vi "Path to Class.vi"(8 "error in (no error)":errorcluster) -> (0 "error out":errorcluster, 3 "Usuarios out":refnum<class "Usuarios.lvclass">)   [LabVIEW 2019, in "Usuarios.lvclass"]
uses:
  Usuarios.lvclass
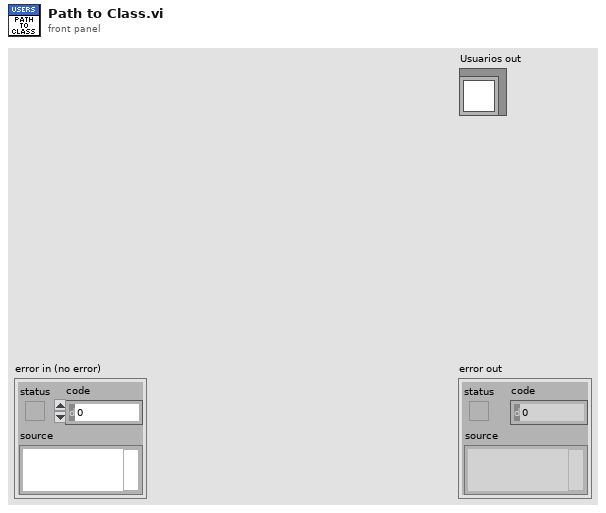
[diagram p1: front panel]
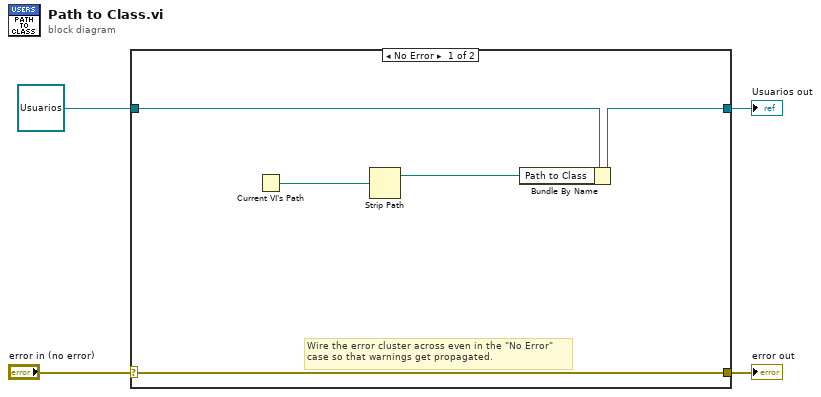
[diagram p0: block diagram]
diagram:
  n1 = case shown="No Error" "error in (no error)" {
    selector: "error in (no error)" -> [w8 w11]
    tunnel: [w8 w11] -> w3
    tunnel: [w6 w10] -> w1
    tunnel: refnum<class "Usuarios.lvclass"> refnum ("Usuarios in") -> [w9 w10]
    frame No Error {
      # "Wire the error cluster across even in the \"No Error\"\ncase so that warnings get propagated."
      n2 = Current VI's Path() -> (path=w7:path)
      n3 = Strip Path(path=w7) -> (stripped path=w5:path)  [unwired: 1 out]
      n4 = Bundle By Name(cluster=w9, "Path to Class"=w5) -> (w6:refnum<class "Usuarios.lvclass">)
    }
    frame Error {
    }
  }
  "error out" <- w3
  "Usuarios out" <- w1
